vi "BSON_bytes_to_U64.vi"(11 "BSONbytes":u8[](array[numeric])) -> (3 "value":u64)   [LabVIEW 2015, in "BSON_convertors_Library.lvlib"]
doc: "Created by Artem Shevelev\nLabVIEW Portal profile: http://www.labviewportal.org/memberlist.php?mode=viewprofile&u=2340\ne-mail: artem.sh@gmail.com\nshevelev.pro"
uses:
  BSON_convertors_Library.lvlib
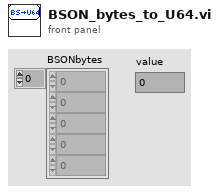
[diagram p1: front panel]
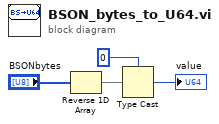
[diagram p0: block diagram]
diagram:
  n1 = Reverse 1D Array(array="BSONbytes") -> (reversed array=w3:u8[])
  n2 = Type Cast(type=u64 0, x=w3) -> (*(type *) &x=→"value":u64)
